vi "Is square occupied.vi"(8 "error in (no error)":errorcluster, 10 "Square":T1={"File"=enum."a", "Rank"=enum."4"}, 11 "Position in":refnum<class "Position.lvclass">) -> (0 "error out":errorcluster, 1 "Piece":refnum<class "Piece.lvclass">, 2 "Occupied":bool, 3 "Position out":refnum<class "Position.lvclass">)   [LabVIEW 2016, in "Chesslib.lvlib" / "Position.lvclass"]
uses:
  Position.lvclass
  typedef/Square.ctl
  typedef/File.ctl
  typedef/Rank.ctl
  Pieces/Piece/Piece.lvclass
  Position.lvclass/Position.ctl
  Board/Board.lvclass
  Chesslib.lvlib
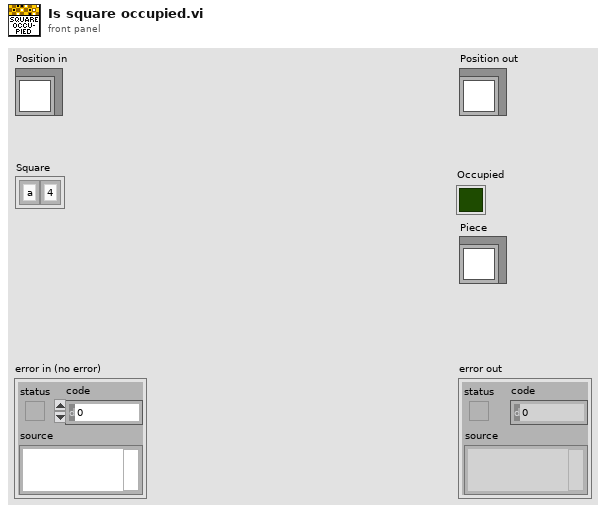
[diagram p1: front panel]
types:
  T1 = typedef "Chesslib.lvlib/Square.ctl" = cluster{"File":T2, "Rank":T3}
  T2 = typedef "Chesslib.lvlib/File.ctl" = enum8{"a", "b", "c", "d", "e", "f", "g", "h"}
  T3 = typedef "Chesslib.lvlib/Rank.ctl" = enum8{"1", "2", "3", "4", "5", "6", "7", "8"}
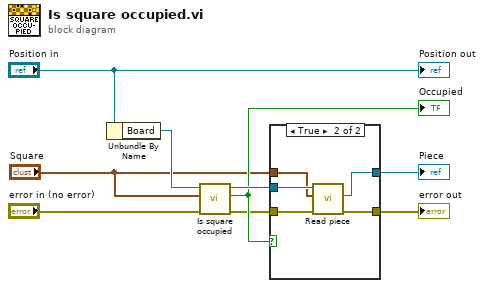
[diagram p0: block diagram]
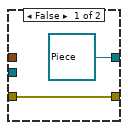
[diagram p2: hidden frame]
diagram:
  n1 = Unbundle By Name("Position in") -> ("Board"=w8:refnum<class "Board.lvclass">)
  n2 = call "Is square occupied.vi"("error in (no error)"="error in (no error)", "Square"="Square", "Board in"=w8) -> ("error out"=w3:errorcluster, "Occupied"=w5:bool, "Board out"=w6:refnum<class "Board.lvclass">)  [unwired: 6 in]
  "Occupied" <- w5
  n3 = case shown="True" w5 {
    tunnel: w6 -> [_ w16]
    tunnel: "Square" -> [_ w15]
    tunnel: w3 -> [w11 w14]
    tunnel: [w11 w13] -> w2
    tunnel: [refnum<class "Piece.lvclass"> refnum ("Piece") w12] -> w1
    frame False {
    }
    frame True {
      n4 = call "Read piece.vi"("error in (no error)"=w14, "Square"=w15, "Board in"=w16) -> ("error out"=w13:errorcluster, "Piece"=w12:refnum<class "Piece.lvclass">)  [unwired: 6 in, 1 out]
    }
  }
  "error out" <- w2
  "Piece" <- w1
  "Position out" <- "Position in"
